vi "Read Pump-B Command.vi"(8 "error in (no error)":errorcluster, 11 "DCM-DSI-HW in":refnum<class "DCM-DSI.lvclass">) -> (0 "error out":errorcluster, 2 "Pump-B Command":T1={"Mode"=enum."Off", "Digital Input"=enum."Unused", "Default Profile Index"=0, "Cal Freq [Hz]"=0.0, "Cal Duration [s]"=0.0, "Cal Increment [s]"=0.0, "Cal Pulses"=0, "TMP Command Sequence"=[{"Duration [s]"=0.0, "Level"=FALSE, "Run/Stop"=FALSE, "Profile Index"=0}, {"Duration [s]"=0.0, "Level"=FALSE, "Run/Stop"=FALSE, "Profile Index"=0}, {"Duration [s]"=0.0, "Level"=FALSE, "Run/Stop"=FALSE, "Profile Index"=0}, {"Duration [s]"=0.0, "Level"=FALSE, "Run/Stop"=FALSE, "Profile Index"=0}, {"Duration [s]"=0.0, "Level"=FALSE, "Run/Stop"=FALSE, "Profile Index"=0}, {"Duration [s]"=0.0, "Level"=FALSE, "Run/Stop"=FALSE, "Profile Index"=0}, {"Duration [s]"=0.0, "Level"=FALSE, "Run/Stop"=FALSE, "Profile Index"=0}, {"Duration [s]"=0.0, "Level"=FALSE, "Run/Stop"=FALSE, "Profile Index"=0}], "EPT TDC Offset [CAD]"=0.0, "EPT Window Start [DBTDC]"=0.0, "EPT Window End [DBTDC]"=0.0, "EPT Angles"=[{"Enable"=FALSE, "Timing [DBTDC]"=0.0, "Duration [s]"=0.0, "Profile Index"=0}, {"Enable"=FALSE, "Timing [DBTDC]"=0.0, "Duration [s]"=0.0, "Profile Index"=0}, {"Enable"=FALSE, "Timing [DBTDC]"=0.0, "Duration [s]"=0.0, "Profile Index"=0}, {"Enable"=FALSE, "Timing [DBTDC]"=0.0, "Duration [s]"=0.0, "Profile Index"=0}], "EPT Skip Fire"=FALSE, "EPT Skip Index"=0, "EPT Precharge Duration [s]"=0.0, "EPT Precharge Profile Index"=0} {"EPT Precharge Profile Index" max=15; "EPT Precharge Duration [s]" min=0 format="%#_4p"; "Default Profile Index" max=15; "Cal Increment [s]" format="%#_3p"; "TMP Command Sequence"."Profile Index" max=7; "TMP Command Sequence"."Duration [s]" min=0 max=100 format="%#_3p"; "Cal Pulses" max=511; "EPT Skip Index" max=7; "EPT Angles"."Profile Index" max=7; "EPT Angles"."Duration [s]" min=0 max=100 format="%#_3p"; "Cal Duration [s]" format="%#_3p"; "Cal Freq [Hz]" format="%#_3p"}, 3 "DCM-DSI-HW out":refnum<class "DCM-DSI.lvclass">)   [LabVIEW 2016, in "DCM-DSI.lvclass"]
uses:
  DCM-DSI.lvclass
  <vilib>/Powertrain Controls/Device Drivers/DCM/DI/RT/Command.ctl
  <vilib>/Powertrain Controls/Device Drivers/DCM/DI/FPGA/Mode.ctl
  <vilib>/Powertrain Controls/Device Drivers/DCM/Rev0/FPGA/Digital Channel.ctl
  <vilib>/Powertrain Controls/Device Drivers/DCM/DI/RT/Command Sequence.ctl
  <vilib>/Powertrain Controls/Device Drivers/DCM/DI/RT/Angle Control.ctl
  DCM-DSI.lvclass/DCM-DSI.ctl
  <vilib>/Powertrain Controls/Device Drivers/DCM/DI/RT/DCM - RT - DI.lvlib
  <vilib>/Powertrain Controls/Device Drivers/DCM/DI/FPGA/DCM - FPGA - DI.lvlib
  <vilib>/Powertrain Controls/Device Drivers/DCM/Rev0/FPGA/DCM - FPGA.lvlib
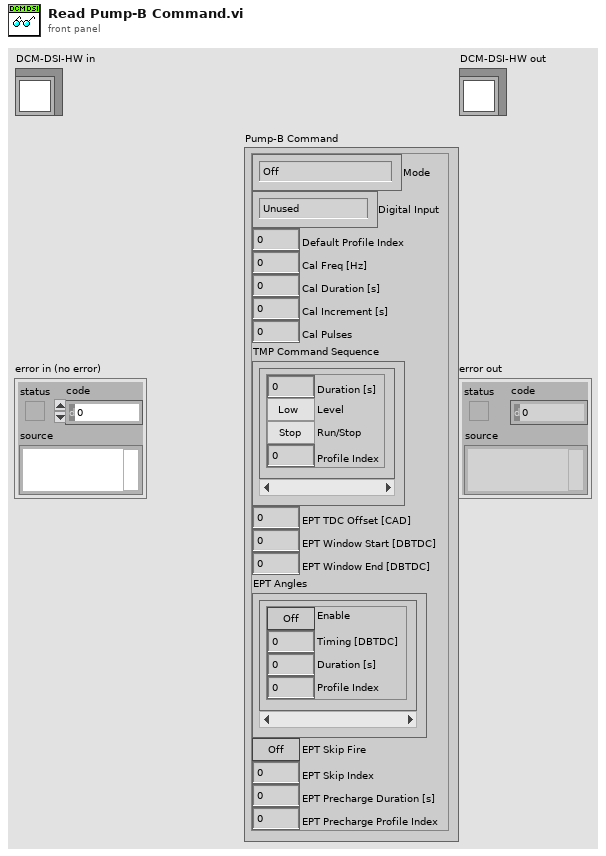
[diagram p1: front panel]
types:
  T1 = typedef "DCM - RT - DI.lvlib/Command.ctl" = cluster{"Mode":T2, "Digital Input":T3, "Default Profile Index":u8, "Cal Freq [Hz]":sgl, "Cal Duration [s]":sgl, "Cal Increment [s]":sgl, "Cal Pulses":u16, "TMP Command Sequence":T4[], "EPT TDC Offset [CAD]":sgl, "EPT Window Start [DBTDC]":sgl, "EPT Window End [DBTDC]":sgl, "EPT Angles":T5[], "EPT Skip Fire":bool, "EPT Skip Index":u8, "EPT Precharge Duration [s]":sgl, "EPT Precharge Profile Index":u8}
  T2 = typedef "DCM - FPGA - DI.lvlib/Mode.ctl" = enum8{"Off", "Direct", "Calibration", "Triggered Multi-Pulse", "Engine Position Tracking"}
  T3 = typedef "DCM - FPGA.lvlib/Digital Channel.ctl" = enum8{"Unused", "User OS", "Diff IO 1", "Diff IO 2", "Diff IO 3", "Diff IO 4", "Diff IO 5", "Diff IO 6", "Diff IO 7", "Diff IO 8", "Aux 1", "Aux 2", "Aux 3", "Aux 4", "Aux 5", "Aux 6", "Aux 7", "Aux 8", "Aux 9", "Aux 10", "Aux 11", "Aux 12", "Aux 13", "Aux 14", "Aux 15", "Aux 16"}
  T4 = typedef "DCM - RT - DI.lvlib/Command Sequence.ctl" = cluster{"Duration [s]":sgl, "Level":bool, "Run/Stop":bool, "Profile Index":u8}
  T5 = typedef "DCM - RT - DI.lvlib/Angle Control.ctl" = cluster{"Enable":bool, "Timing [DBTDC]":sgl, "Duration [s]":sgl, "Profile Index":u8}
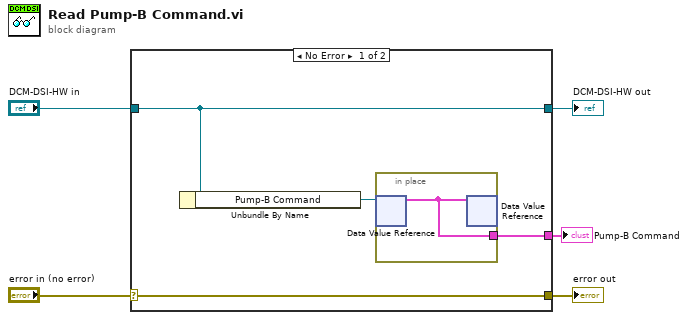
[diagram p0: block diagram]
diagram:
  n1 = case shown="No Error" "error in (no error)" {
    selector: "error in (no error)" -> [w9 w12]
    tunnel: [w9 w12] -> w4
    tunnel: [w7 w11] -> w2
    tunnel: "DCM-DSI-HW in" -> [w7 w11]
    tunnel: [w6 _] -> w1
    frame No Error {
      n2 = Unbundle By Name(w7) -> ("Pump-B Command"=w8:refnum<data-value>)
      n3 = in-place {
        in-place-border: [w10] -> w6
        n4 = in-place-dvr #1(w8) -> (w10:T1)  [unwired: 1 out]
        n5 = in-place-dvr #1(w10) -> ()  [unwired: 2 out]
      }
    }
    frame Error {
    }
  }
  "error out" <- w4
  "DCM-DSI-HW out" <- w2
  "Pump-B Command" <- w1
